vi "CalculateMerit.vi"(7 "RangeInfo":T1, 9 "idealSPFraction":dbl=0.7 format="%#_13g", 10 "Target":dbl, 11 "MeritMeasure":enum16{"MinMFCs", "ClosestToIdeal", "Weighted"}(ring)=enum."ClosestToIdeal") -> (0 "Merit (smaller is better)":dbl, 1 "OffsetFromIdeal":dbl, 2 "LocationInRange":dbl, 3 "In Range?":bool)   [LabVIEW 2018]
uses:
  ComboRange.ctl
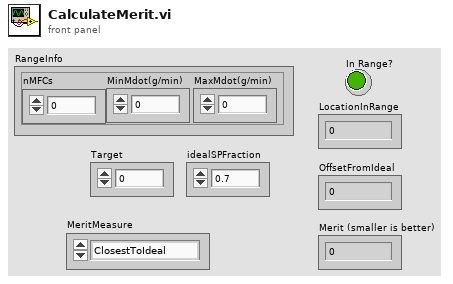
[diagram p1: front panel]
types:
  T1 = typedef "ComboRange.ctl" = cluster{"nMFCs":i32, "MinMdot(g/min)":dbl, "MaxMdot(g/min)":dbl}
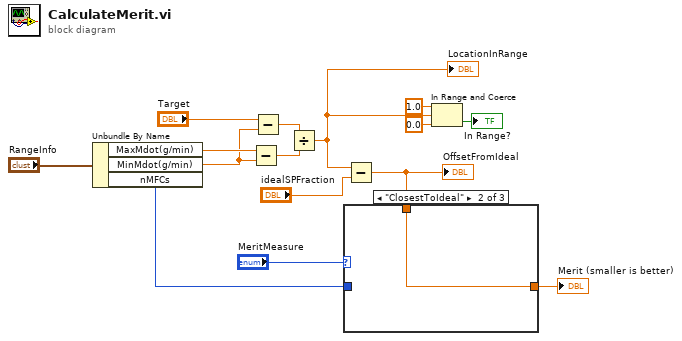
[diagram p0: block diagram]
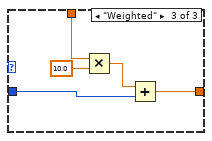
[diagram p3: hidden frame]
diagram:
  n1 = Unbundle By Name("RangeInfo") -> ("MaxMdot(g/min)"=w6:dbl, "MinMdot(g/min)"=w5:dbl, "nMFCs"=w4:i32)
  n2 = Subtract(x=w6, y=w5) -> (x-y=w14:dbl)
  n3 = Subtract(x="Target", y=w5) -> (x-y=w13:dbl)
  n4 = Divide(x=w13, y=w14) -> (x/y=w12:dbl)
  "LocationInRange" <- w12
  n5 = Subtract(x=w12, y="idealSPFraction") -> (x-y=w2:dbl)
  "OffsetFromIdeal" <- w2
  n6 = case shown="\"ClosestToIdeal\"" "MeritMeasure" {
    tunnel: w4 -> [w16 _ w21]
    tunnel: w2 -> [_ w17 w19]
    tunnel: [w16 w17 w18] -> w1
    frame "MinMFCs", Default {
    }
    frame "ClosestToIdeal" {
    }
    frame "Weighted" {
      n7 = Multiply(x=w19, y=10.0) -> (x*y=w22:dbl)
      n8 = Add(x=w22, y=w21) -> (x+y=w18:dbl)
    }
  }
  "Merit (smaller is better)" <- w1
  n9 = In Range and Coerce(upper limit=1.0, x=w12, lower limit=0.0) -> (In Range?=→"In Range?":bool)  [unwired: 1 out]
